vi "CloseServerHandles.vi"(0 "ROS":T1={"topic port"=0, "Node"="", "topic"="", "type"="", "node port"=0, "error "={"status"=FALSE, "code"=0, "source"=""}, "Direction"=enum."Node", "APIs"=[], "Update (ms)"=1, "write queue"=1}) -> ()   [LabVIEW 2010]
uses:
  SubVIs/_ROSDirection.ctl
  SubVIs/_ROSControl.ctl
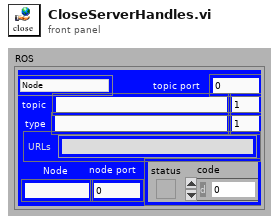
[diagram p1: front panel]
types:
  T1 = typedef "_ROSControl.ctl" = cluster{"topic port":u16, "Node":string, "topic":string, "type":string, "node port":u32, "error ":errorcluster, "Direction":T2, "APIs":string[], "Update (ms)":u16, "write queue":u16}
  T2 = typedef "_ROSDirection.ctl" = enum16{"Node", "Publisher", "Subscriber", "Service Client"}
  T3 = enum16{"Add Server", "Clear Server", "Clear All", "Get Info"}
  T4 = typedef "ServoInfo.ctl" = cluster{"vi name":string, "VI Refnum":refnum<vi>, "queue":refnum<queue>, "ROS":T1, "notifier":refnum<notifier>}
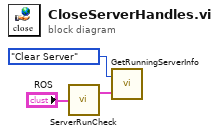
[diagram p0: block diagram]
diagram:
  n1 = call "ServerRunCheck.vi"("ROS in"="ROS") -> ("ServerFound"=w1:T4)  [unwired: 1 out]
  n2 = call "GetRunningServerInfo.vi"("New Server"=w1, "Task"=T3."Clear Server") -> ()  [unwired: 3 out]
